vi "Read Compatible Hardware Types.vi"(8 "error in (no error)":errorcluster, 11 "Standard Measurement in":refnum<class "Standard Measurement.lvclass">) -> (0 "error out":errorcluster, 2 "Compatible Hardware Types":string[](array[string]), 3 "Standard Measurement out":refnum<class "Standard Measurement.lvclass">)   [LabVIEW 2026, in "Standard Measurement Plugin.lvlib" / "Standard Measurement.lvclass"]
uses:
  Standard Measurement.lvclass
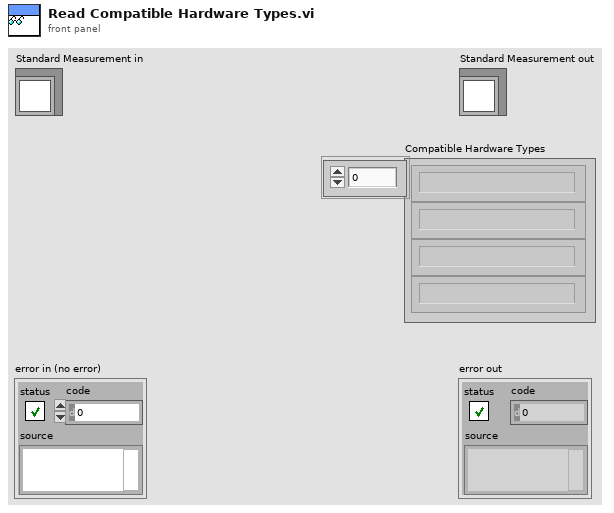
[diagram p1: front panel]
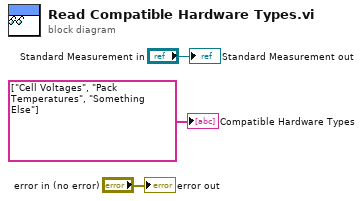
[diagram p0: block diagram]
diagram:
  "error out" <- "error in (no error)"
  "Standard Measurement out" <- "Standard Measurement in"
  "Compatible Hardware Types" <- string[] ["Cell Voltages", "Pack Temperatures", "Something Else"] ("Compatible Hardware Types")
